vi "Example.vi"() -> ()   [LabVIEW 2025]
uses:
  ObserverClass/ObserverClass.lvclass
  dc965987-80da-45ca-bf8e-831b3f56a045.vi
  messages/NotifyObserver_Array.vi
  messages/NotifyObserver_Single.vi
  messages/NotifyObserver_Container.vi
  ObserverClass.lvlib
panel:
  out "Obs2-IsSender":bool
  out "Obs1-IsSender":bool
  out "obs2":T1(array[cluster])
  out "obs1":T1(array[cluster])
  in  "stop":bool
  # "Observer Pattern Example Description\nThis example demonstrates how to easily implement the Observer pattern in LabVIEW using a dedicated Observer class.\nThe demo creates two independent Observer instances, each registered to specific Observable data sources. \nWhenever the Observables change, they trigger updates through the NotifyObserver method, \nensuring that each Observer instance receives and processes the latest data automatically.\n\nThis example provides a clean and scalable approach to event-driven communication between objects in LabVIEW, \nmaking it ideal for modular architectures, UI updates, or decoupled data monitoring systems."
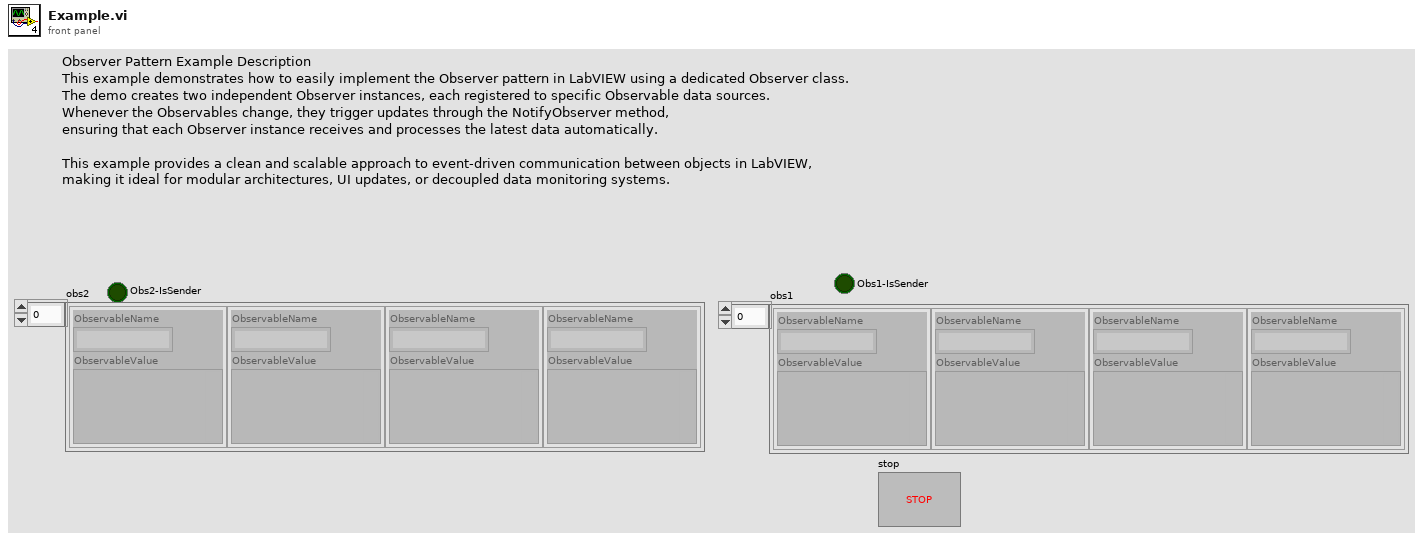
[diagram p1: front panel]
types:
  T1 = cluster{"ObservableName":string, "ObservableValue":variant}[]
  T2 = enum8{"Enabled", "Disabled", "Disabled and Grayed Out"}
  T3 = cluster{"ObservableName":string, "ObservableValue":variant}
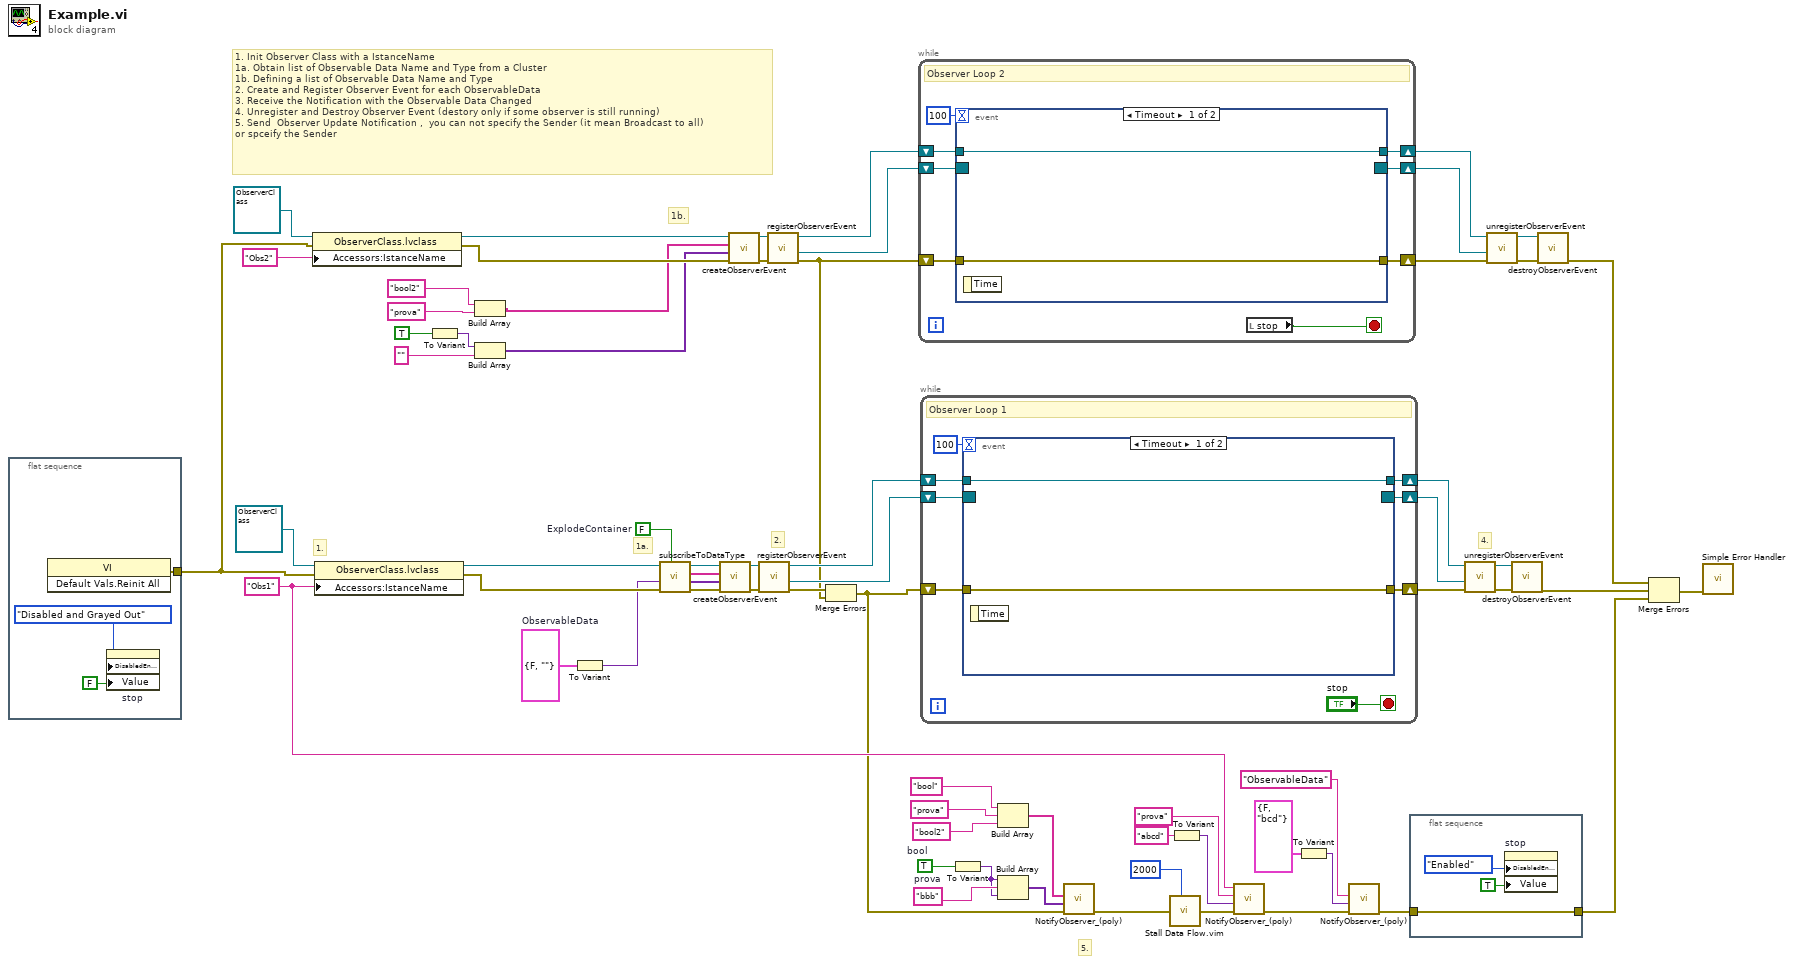
[diagram p0: block diagram]
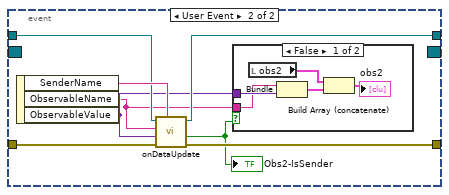
[diagram p2: hidden frame]
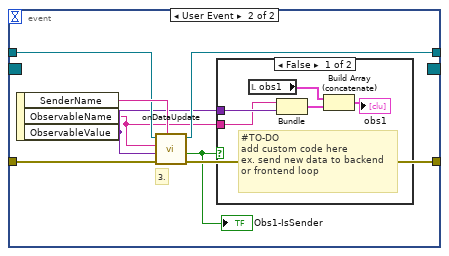
[diagram p4: hidden frame]
diagram:
  w1 = FALSE  # ExplodeContainer
  w50 = "bbb"  # prova
  w49 = TRUE  # bool
  w51 = cluster{"bool":bool, "prova":string} {"bool"=FALSE, "prova"=""}  # ObservableData
  w27 = "Obs1" ("IstanceName")
  # "1b."
  # "1a."
  # "1. Init Observer Class with a IstanceName\n1a. Obtain list of Observable Data Name and Type from a Cluster\n1b. Defining a list of Observable Data Name and Type\n2. Create and Register Observer Event for each ObservableData\n3. Receive the Notification with the Observable Data Changed\n4. Unregister and Destroy Observer Event (destory only if some observer is still running)\n5. Send  Observer Update Notification ,  you can not specify the Sender (it mean Broadcast to all)\nor spceify the Sender"
  # "5."
  # "4."
  # "2."
  # "1."
  n1 = flat-sequence {
    tunnel: [w70] -> w18
    frame #0 {
      n2 = invoke class="VI" method="Default Vals.Reinit All"() -> (error out=w70:errorcluster)  [unwired: 3 in, 2 out]
      n3 = property on="stop" class="Bool (strict)"("DisabledEnum"=T2."Disabled and Grayed Out" ("Disabled"), "Value"=FALSE ("stop")) -> ()  [unwired: 2 in, 2 out]
    }
  }
  n4 = property class="ObserverClass.lvclass"(reference=refnum<class "ObserverClass.lvclass"> refnum ("ObserverClass in"), error in=w18, "Accessors:IstanceName"="Obs2" ("IstanceName")) -> (reference out=w43:refnum<class "ObserverClass.lvclass">, error out=w45:errorcluster)
  n5 = property class="ObserverClass.lvclass"(reference=refnum<class "ObserverClass.lvclass"> refnum ("ObserverClass in"), error in=w18, "Accessors:IstanceName"=w27) -> (reference out=w53:refnum<class "ObserverClass.lvclass">, error out=w52:errorcluster)
  n6 = To Variant(anything=TRUE ("bool")) -> (Variant=w14:variant)
  n7 = Build Array("bool2" ("prova"), "prova" ("prova")) -> (w13:string[])
  n8 = Build Array(w14, "" ("prova")) -> (w11:variant[])
  n9 = To Variant(anything=w51) -> (Variant=w10:variant)
  n10 = call-dynamic "subscribeToDataType.vi"("ExplodeContainer (F)"=w1, "error in"=w52, "ObservableData"=w10, "ObserverClass in"=w53) -> ("error out"=w67:errorcluster, "ObservableValue"=w61:variant[], "ObservableName"=w60:string[], "ObserverClass out"=w66:refnum<class "ObserverClass.lvclass">)  [unwired: 4 in]
  n11 = call-dynamic "createObserverEvent.vi"("error in"=w67, "ObservableValue"=w61, "ObservableName"=w60, "ObserverClass in"=w66) -> ("error out"=w62:errorcluster, "ObserverClass out"=w65:refnum<class "ObserverClass.lvclass">)  [unwired: 5 in, 1 out]
  n12 = call-dynamic "createObserverEvent.vi"("error in"=w45, "ObservableValue"=w11, "ObservableName"=w13, "ObserverClass in"=w43) -> ("error out"=w36:errorcluster, "ObserverClass out"=w33:refnum<class "ObserverClass.lvclass">)  [unwired: 5 in, 1 out]
  n13 = call-dynamic "registerObserverEvent.vi"("error in"=w62, "ObserverClass in"=w65) -> ("error out"=w6:errorcluster, "EventReg"=w58:refnum<event-registration>, "ObserverClass out"=w55:refnum<class "ObserverClass.lvclass">)  [unwired: 6 in, 1 out]
  n14 = call-dynamic "registerObserverEvent.vi"("error in"=w36, "ObserverClass in"=w33) -> ("error out"=w4:errorcluster, "EventReg"=w38:refnum<event-registration>, "ObserverClass out"=w41:refnum<class "ObserverClass.lvclass">)  [unwired: 6 in, 1 out]
  n15 = Merge Errors(w6, w4) -> (w3:errorcluster)
  n16 = while {
    shift-right: [w75] -> w40
    shift-left: w4 -> [w78]
    shift-right: [w76] -> w39
    shift-left: w38 -> [w77]
    shift-right: [w72] -> w42
    shift-left: w41 -> [w73]
    stop <- w71 stop-if-true
    # "Observer Loop 2"
    n17 = event shown="[0] Timeout" {
      selector: w77 -> [_ _]
      dyn-events: [_ _] -> w76
      timeout: 100 -> [_ _]
      tunnel: w78 -> [w80 w88]
      tunnel: [w80 w86] -> w75
      tunnel: w73 -> [w79 w84]
      tunnel: [w79 w85] -> w72
      event Timeout {
        n18 = event-data() -> ()  [unwired: 1 in, 1 out]
      }
      event User Event {
        n19 = event-data() -> ("SenderName"=w87:string, "ObservableName"=w82:string, "ObservableValue"=w83:variant)  [unwired: 1 in]
        n20 = call-dynamic "onDataUpdate.vi"("SenderName"=w87, "error in"=w88, "ObservableValue"=w83, "ObservableName"=w82, "ObserverClass in"=w84) -> ("error out"=w86:errorcluster, "IsSender"=w81:bool, "ObserverClass out"=w85:refnum<class "ObserverClass.lvclass">)  [unwired: 4 in]
        "Obs2-IsSender" <- w81
        n21 = case shown="False" w81 {
          tunnel: w83 -> [w93 _]
          tunnel: w82 -> [w92 _]
          frame False {
            n22 = local read "obs2"() -> (w89:T1)
            n23 = Bundle("ObservableName"=w92, "ObservableValue"=w93) -> (w91:T3)  [unwired: 1 in]
            n24 = Build Array (concatenate)(w89, w91) -> (→"obs2":T1)
          }
          frame True {
          }
        }
      }
    }
    n25 = local read "stop"() -> (w71:bool)
  }
  n26 = while {
    shift-right: [w98] -> w56
    shift-left: w3 -> [w101]
    shift-right: [w99] -> w57
    shift-left: w58 -> [w100]
    shift-right: [w94] -> w54
    shift-left: w55 -> [w95]
    stop <- "stop" stop-if-true
    # "Observer Loop 1"
    n27 = event shown="[0] Timeout" {
      selector: w100 -> [_ _]
      dyn-events: [_ _] -> w99
      timeout: 100 -> [_ _]
      tunnel: w101 -> [w103 w111]
      tunnel: [w103 w109] -> w98
      tunnel: w95 -> [w102 w107]
      tunnel: [w102 w108] -> w94
      event Timeout {
        n28 = event-data() -> ()  [unwired: 1 in, 1 out]
      }
      event User Event {
        # "3."
        n29 = event-data() -> ("SenderName"=w110:string, "ObservableName"=w105:string, "ObservableValue"=w106:variant)  [unwired: 1 in]
        n30 = call-dynamic "onDataUpdate.vi"("SenderName"=w110, "error in"=w111, "ObservableValue"=w106, "ObservableName"=w105, "ObserverClass in"=w107) -> ("error out"=w109:errorcluster, "IsSender"=w104:bool, "ObserverClass out"=w108:refnum<class "ObserverClass.lvclass">)  [unwired: 4 in]
        "Obs1-IsSender" <- w104
        n31 = case shown="False" w104 {
          tunnel: w106 -> [w116 _]
          tunnel: w105 -> [w115 _]
          frame False {
            # "#TO-DO\nadd custom code here\nex. send new data to backend\nor frontend loop"
            n32 = local read "obs1"() -> (w112:T1)
            n33 = Bundle("ObservableName"=w115, "ObservableValue"=w116) -> (w114:T3)  [unwired: 1 in]
            n34 = Build Array (concatenate)(w112, w114) -> (→"obs1":T1)
          }
          frame True {
          }
        }
      }
    }
  }
  n35 = To Variant(anything=w49) -> (Variant=w31:variant)
  n36 = Build Array("bool" ("prova"), "prova" ("prova"), "bool2" ("prova")) -> (w29:string[])
  n37 = Build Array(w31, w50, w31) -> (w46:variant[])
  n38 = call-poly "NotifyObserver_(poly).vi"("error in"=w3, "ObservableDataValue"=w46, "ObservableDataName"=w29) -> ("error out"=w30:errorcluster)  [unwired: 8 in]
  n39 = call "Stall Data Flow.vim"("value in"=w30, "milliseconds to wait"=u32 2000) -> ("value out"=w24:errorcluster)  [unwired: 1 out]
  n40 = To Variant(anything="abcd" ("prova")) -> (Variant=w28:variant)
  n41 = call-poly "NotifyObserver_(poly).vi"("error in"=w24, "ObservableDataValue"=w28, "ObservableDataName"="prova" ("prova"), "IstanceName"=w27) -> ("error out"=w7:errorcluster)  [unwired: 7 in]
  n42 = To Variant(anything=cluster{"bool":bool, "prova":string} {"bool"=FALSE, "prova"="bcd"} ("ObservableData")) -> (Variant=w8:variant)
  n43 = call-poly "NotifyObserver_(poly).vi"("error in"=w7, "ObservableDataValue"=w8, "ObservableDataName"="ObservableData" ("prova")) -> ("error out"=w5:errorcluster)  [unwired: 8 in]
  n44 = flat-sequence {
    tunnel: w5 -> [w119]
    tunnel: [w119] -> w19
    frame #0 {
      n45 = property on="stop" class="Bool (strict)"("DisabledEnum"=T2."Enabled" ("Disabled"), "Value"=TRUE ("stop")) -> ()  [unwired: 2 in, 2 out]
    }
  }
  n46 = call-dynamic "unregisterObserverEvent.vi"("error in"=w56, "EventReg"=w57, "ObserverClass in"=w54) -> ("error out"=w63:errorcluster, "ObserverClass out"=w64:refnum<class "ObserverClass.lvclass">)  [unwired: 7 in]
  n47 = call-dynamic "unregisterObserverEvent.vi"("error in"=w40, "EventReg"=w39, "ObserverClass in"=w42) -> ("error out"=w35:errorcluster, "ObserverClass out"=w34:refnum<class "ObserverClass.lvclass">)  [unwired: 7 in]
  n48 = call-dynamic "destroyObserverEvent.vi"("error in"=w63, "ObserverClass in"=w64) -> ("error out"=w22:errorcluster)  [unwired: 8 in, 1 out]
  n49 = call-dynamic "destroyObserverEvent.vi"("error in"=w35, "ObserverClass in"=w34) -> ("error out"=w21:errorcluster)  [unwired: 8 in, 1 out]
  n50 = Merge Errors(w21, w22, w19) -> (w20:errorcluster)
  n51 = call <vilib>:"Simple Error Handler.vi"("error in (no error)"=w20) -> ()  [unwired: 4 in, 5 out]
